vi "NI-XNET Monitor Start.vi"(8 "Error In":errorcluster, 11 "Process  Data In":T1) -> (0 "Error Out":errorcluster, 3 "Process  Data Out":T1)   [LabVIEW 2017, in "NI-XNET Monitor Engine.lvlib"]
uses:
  NI-XNET Monitor Engine.lvlib
  RTMonitorRefnums.ctl
  <vilib>/NI/NIVS Inline Async API/_Data Access Engine/Data Access Engine/Types/Write.DVR.ctl
  <vilib>/NI/NIVS Inline Async API/_Data Access Engine/Access Type Classes/Write/Write.lvclass
  <vilib>/xnet/xnet.llb/XNET Control Scope.ctl
  <vilib>/NI VeriStand/Custom Device Tools/Custom Device Utility Library/Custom Device Utility Library.lvlib
  <vilib>/NI/NIVS Inline Async API/_Data Access Engine/Data Access Engine/Data Access Engine.lvclass
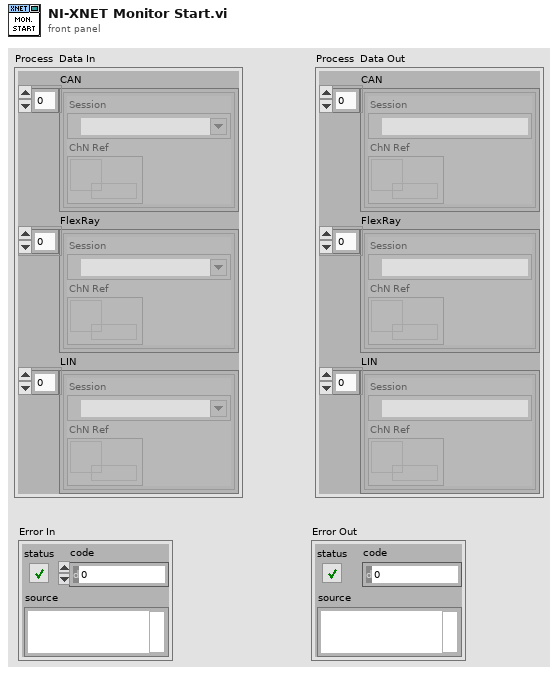
[diagram p1: front panel]
types:
  T1 = typedef "NI-XNET Monitor Engine.lvlib/RTMonitorRefnums.ctl" = cluster{"CAN":cluster{"Session":refnum<k21>, "ChN Ref":T2}[], "FlexRay":cluster{"Session":refnum<k21>, "ChN Ref":T2}[], "LIN":cluster{"Session":refnum<k21>, "ChN Ref":T2}[]}
  T2 = typedef "Data Access Engine.lvlib/Data Access Engine.lvclass/Write.DVR.ctl" = refnum<data-value>
  T3 = typedef "XNET Control Scope.ctl" = u32
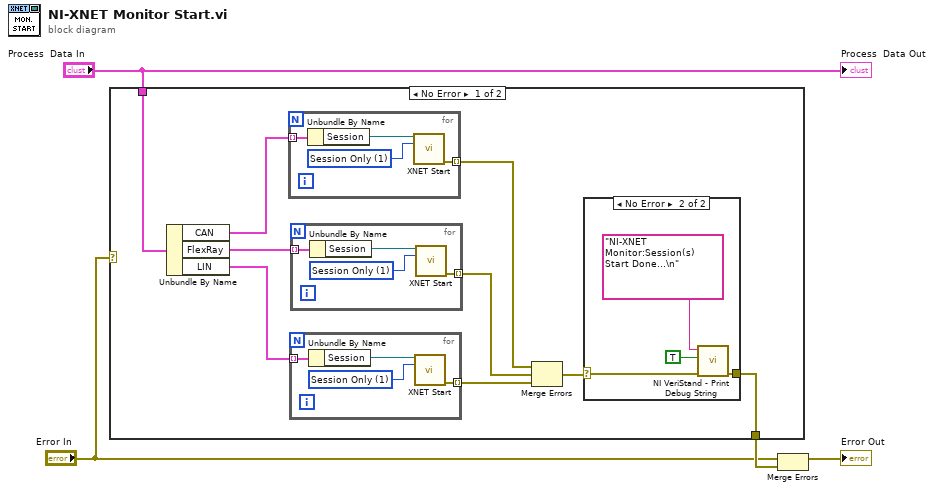
[diagram p0: block diagram]
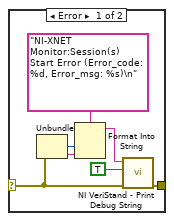
[diagram p2: hidden frame]
diagram:
  n1 = case shown="No Error" "Error In" {
    tunnel: "Process  Data In" -> [w13 _]
    tunnel: [w5 _] -> w2
    frame No Error {
      n2 = Unbundle By Name(w13) -> ("CAN"=w12:cluster{"Session":refnum<k21>, "ChN Ref":T2}[], "FlexRay"=w11:cluster{"Session":refnum<k21>, "ChN Ref":T2}[], "LIN"=w10:cluster{"Session":refnum<k21>, "ChN Ref":T2}[])
      n3 = for {
        tunnel: w12 -> [w36] mode=indexing
        tunnel: [w33] -> w9 mode=indexing
        w34 = T3 1 items=["Normal", "Session Only", "Interface Only", "Session Only Blocking"] ("scope (normal)")
        n4 = Unbundle By Name(w36) -> ("Session"=w35:refnum<k21>)
        n5 = call <vilib>:"XNET Start.vi"("session in"=w35, "scope (normal)"=w34) -> ("error out"=w33:errorcluster)  [unwired: 12 in, 1 out]
      }
      n6 = for {
        tunnel: w10 -> [w28] mode=indexing
        tunnel: [w25] -> w7 mode=indexing
        w26 = T3 1 items=["Normal", "Session Only", "Interface Only", "Session Only Blocking"] ("scope (normal)")
        n7 = Unbundle By Name(w28) -> ("Session"=w27:refnum<k21>)
        n8 = call <vilib>:"XNET Start.vi"("session in"=w27, "scope (normal)"=w26) -> ("error out"=w25:errorcluster)  [unwired: 12 in, 1 out]
      }
      n9 = for {
        tunnel: w11 -> [w32] mode=indexing
        tunnel: [w29] -> w8 mode=indexing
        w30 = T3 1 items=["Normal", "Session Only", "Interface Only", "Session Only Blocking"] ("scope (normal)")
        n10 = Unbundle By Name(w32) -> ("Session"=w31:refnum<k21>)
        n11 = call <vilib>:"XNET Start.vi"("session in"=w31, "scope (normal)"=w30) -> ("error out"=w29:errorcluster)  [unwired: 12 in, 1 out]
      }
      n12 = Merge Errors(w9, w8, w7) -> (w6:errorcluster)
      n13 = case shown="No Error" w6 {
        selector: w6 -> [w15 w23]
        tunnel: [w14 w22] -> w5
        frame Error {
          n14 = Unbundle(w15) -> ("code"=w19:i32, "source"=w20:string)  [unwired: 1 out]
          n15 = Format Into String(format string="NI-XNET Monitor:Session(s) Start Error (Error_code: %d, Error_msg: %s)\n" ("Message"), w19, w20) -> (resulting string=w18:string)  [unwired: 2 in, 1 out]
          n16 = call <vilib>:"NI VeriStand - Print Debug String.vi"("error in (no error)"=w15, "Add to log file? (T)"=TRUE, "Message"=w18) -> ("error out"=w14:errorcluster)  [unwired: 8 in]
        }
        frame No Error {
          n17 = call <vilib>:"NI VeriStand - Print Debug String.vi"("error in (no error)"=w23, "Add to log file? (T)"=TRUE, "Message"="NI-XNET Monitor:Session(s) Start Done...\n") -> ("error out"=w22:errorcluster)  [unwired: 8 in]
        }
      }
    }
    frame Error {
    }
  }
  n18 = Merge Errors("Error In", w2) -> (→"Error Out":errorcluster)
  "Process  Data Out" <- "Process  Data In"
